vi "mks670_get_pressure.vi"() -> ()   [LabVIEW 2019]
panel:
  out "Over/Under range?":string
  out "Status":string
  in  "tpg361_visa 3":refnum<visa-resource-name>
  in  "err_in 2":errorcluster
  out "Overall Status":bool
  out "Pressure":string
  out "err_out":errorcluster
  out "tpg361_visa 2":refnum<visa-resource-name>
  in  "tpg361_b2r 2":u32
  in  "tpg361_delay 3":u32=500
  # "Status Notes:\n@ = Valid\n> = Parameter is unrecognized\n? = Invalid data field value\n= Inappropriate command"
  # "\" = Underranged\n# = Overranged\n! = Calibrating"
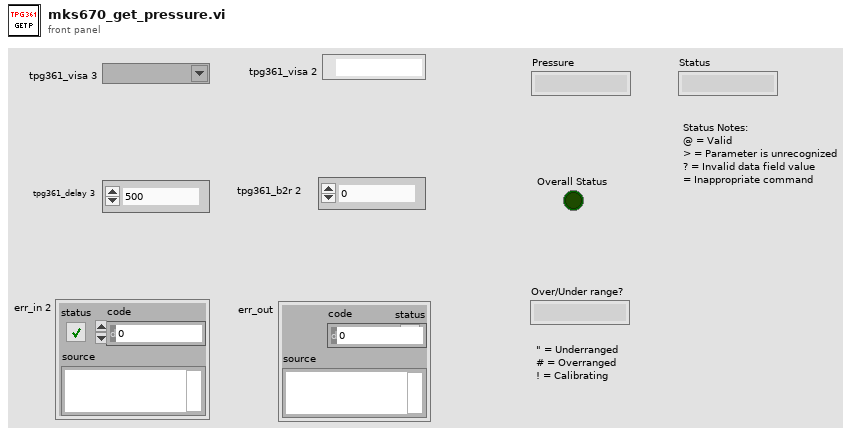
[diagram p1: front panel]
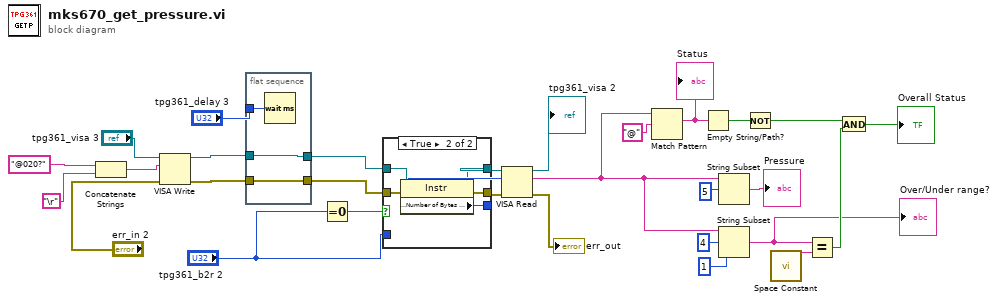
[diagram p0: block diagram]
diagram:
  n1 = Concatenate Strings("@020?" ("write buffer"), "\r") -> (w11:string)
  n2 = VISA Write(VISA resource name="tpg361_visa 3", write buffer=w11, error in (no error)="err_in 2") -> (VISA resource name out=w24:refnum<visa-resource-name>, error out=w23:errorcluster)  [unwired: 1 out]
  n3 = flat-sequence {
    tunnel: [w32] -> w30
    tunnel: [w33] -> w29
    tunnel: w24 -> [w33]
    tunnel: w23 -> [w32]
    tunnel: "tpg361_delay 3" -> [w31]
    frame #0 {
      n4 = Wait (ms)(milliseconds to wait=w31) -> ()  [unwired: 1 out]
    }
  }
  n5 = Equal To 0?(x="tpg361_b2r 2") -> (x = 0?=w28:bool)
  n6 = case shown="True" w28 {
    tunnel: w30 -> [w35 w41]
    tunnel: w29 -> [w36 w40]
    tunnel: [w36 w39] -> w27
    tunnel: [w35 w38] -> w26
    tunnel: [w34 w37] -> w25
    tunnel: "tpg361_b2r 2" -> [w34 _]
    frame False {
    }
    frame True {
      n7 = property class="Instr"(reference=w40, error in=w41) -> (reference out=w39:refnum<visa-resource-name>, error out=w38:errorcluster, "Serial Settings:Number of Bytes at Serial Port"=w37:u32)
    }
  }
  n8 = VISA Read(VISA resource name=w27, byte count=w25, error in (no error)=w26) -> (VISA resource name out=→"tpg361_visa 2":refnum<visa-resource-name>, read buffer=w8:string, error out=→"err_out":errorcluster)  [unwired: 1 out]
  n9 = Match Pattern(string=w8, regular expression="@") -> (match substring=w15:string)  [unwired: 1 in, 3 out]
  "Status" <- w15
  n10 = Empty String/Path?(string/path=w15) -> (empty?=w14:bool)
  n11 = String Subset(string=w8, offset (0)=5) -> (substring=→"Pressure":string)  [unwired: 1 in]
  n12 = String Subset(string=w8, offset (0)=4, length (rest)=1 ("length (rest)")) -> (substring=w1:string)
  "Over/Under range?" <- w1
  n13 = Not(x=w14) -> (.not. x?=w4:bool)
  n14 = call <vilib>:"Space Constant.vi"() -> ("String"=w5:string)
  n15 = Equal?(x=w1, y=w5) -> (x = y?=w3:bool)
  n16 = And(x=w4, y=w3) -> (x .and. y?=→"Overall Status":bool)
